vi "demo_LabVIEW in Linux Docker.vi"(11 "Stop Demo":refnum<user-event>) -> ()   [LabVIEW 2020]
panel:
  # "LabVIEW 2025 Q3 - LabVIEW in a Linux Docker Container\n\nComing later in 2025! We will publish a Docker image that makes it fast and easy to run LabVIEW for Linux in a Docker Container, which is often needed for effective pipelines in CI/CD."
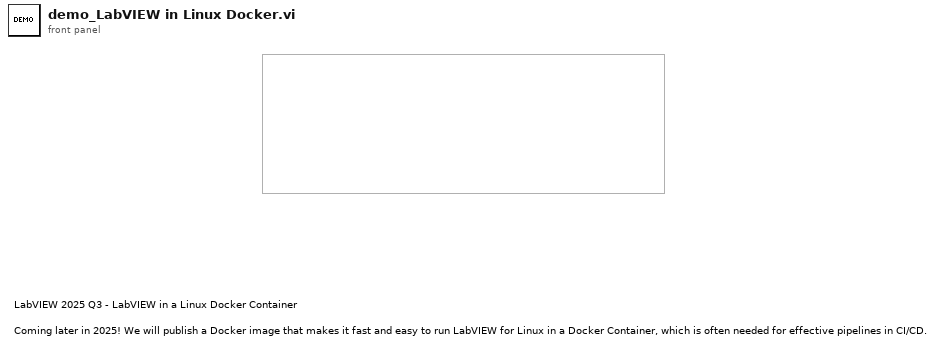
[diagram p1: front panel]
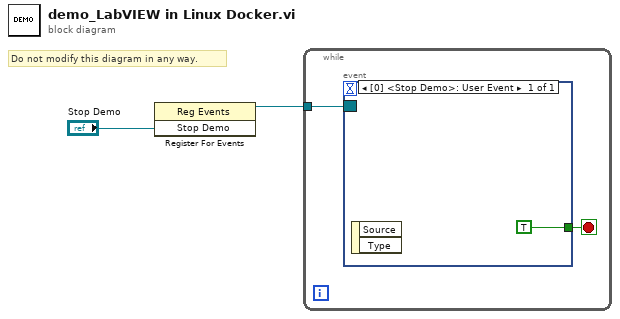
[diagram p0: block diagram]
diagram:
  # "Do not modify this diagram in any way."
  n1 = register-events("Stop Demo") -> (reference out=w1:refnum<event-registration>)  [unwired: 2 in, 1 out]
  n2 = while {
    tunnel: w1 -> [w4]
    stop <- w3 stop-if-true
    n3 = event shown="[0] <Stop Demo>: User Event" {
      selector: w4 -> [_]
      dyn-events: _ -> [_]
      timeout: _ -> [_]
      tunnel: [TRUE] -> w3
      event User Event {
        n4 = event-data() -> ()  [unwired: 1 in, 2 out]
      }
    }
  }
